vi "read big txt.vi"() -> (2 "selected path":path caption="선택된 경로", 3 "Output":string)   [LabVIEW 2015]
panel:
  out "Output 4":string
  out "Output 3":string
  out "Output 2":string
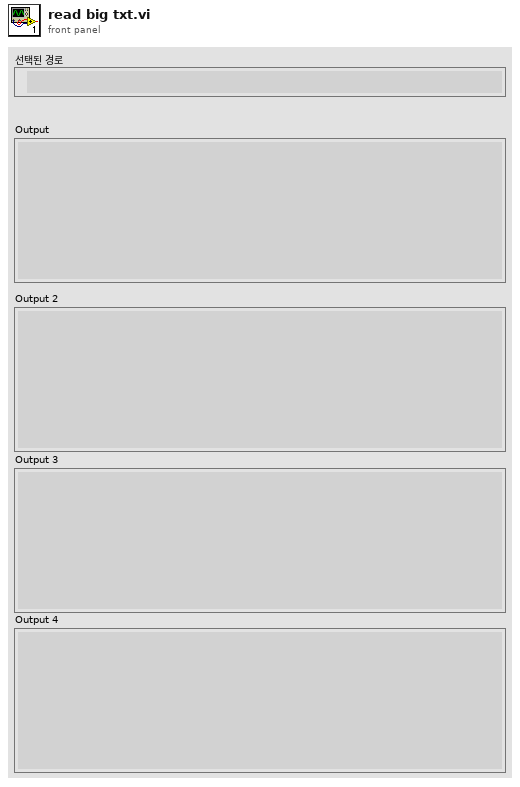
[diagram p1: front panel]
types:
  T1 = enum16{"open", "replace", "create", "open or create", "replace or create", "replace or create with confirmation"}
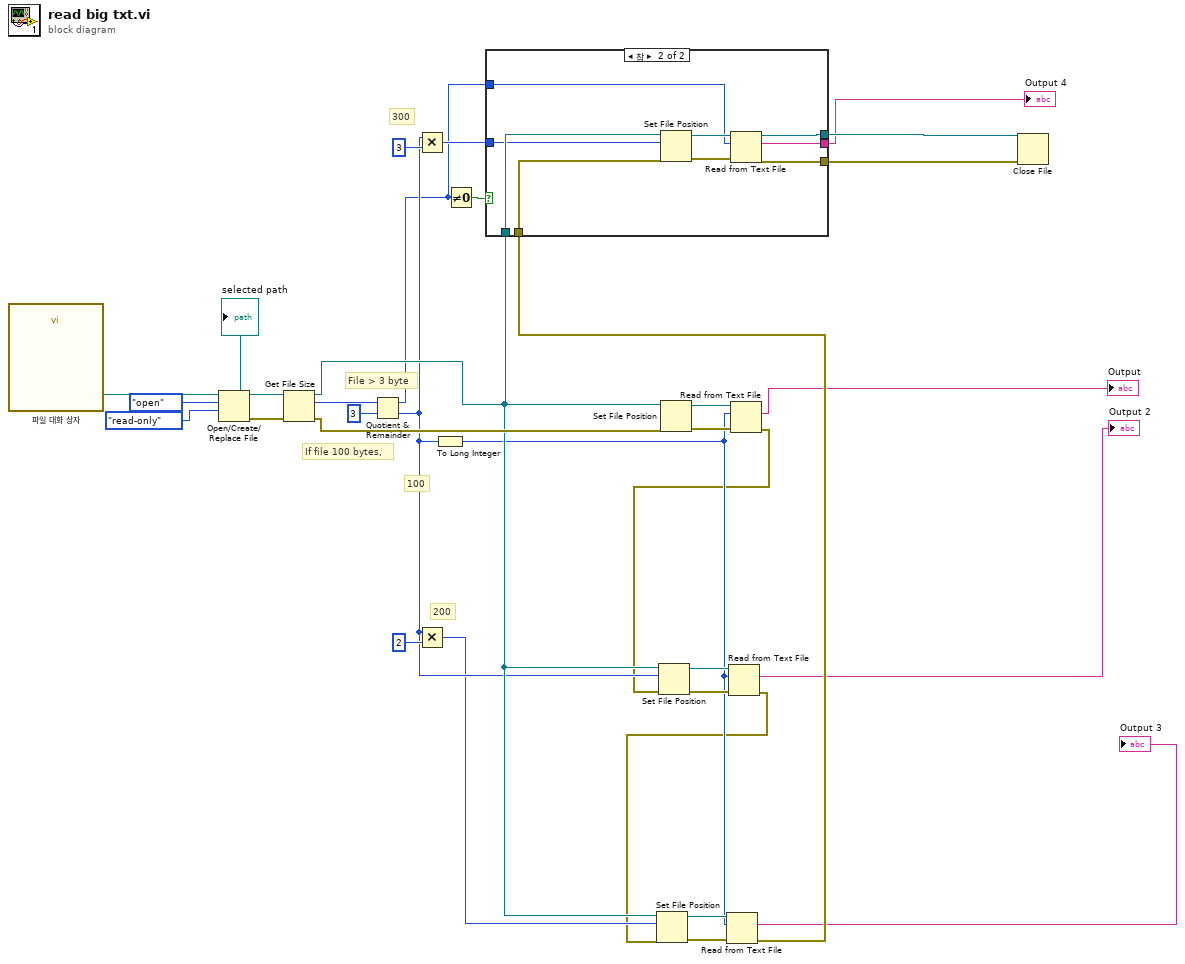
[diagram p0: block diagram]
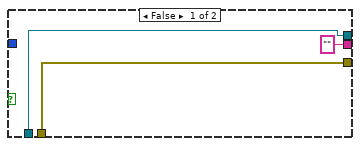
[diagram p2: hidden frame]
diagram:
  # "300"
  # "200"
  # "100"
  # "If file 100 bytes,"
  # "File > 3 byte"
  n1 = call "파일 대화 상자"() -> ("selected path"=w32:path)  [unwired: 12 in, 3 out]
  "selected path" <- w32
  n2 = Open/Create/Replace File(file path (use dialog)=w32, operation (0:open)=T1."open" ("동작(0:open)"), access (0:read/write)=enum16{"read/write", "read-only", "write-only"}."read-only" ("접근(0:읽기/쓰기)")) -> (refnum out=w29:refnum<file>, error out=w28:errorcluster)  [unwired: 3 in, 1 out]
  n3 = Get File Size(file=w29, error in=w28) -> (refnum out=w21:refnum<file>, size (in bytes)=w27:i64, 0:w22:errorcluster)
  n4 = Quotient & Remainder(x=w27, y=i64 3) -> (x-y*floor(x/y)=w10:i64, floor(x/y)=w12:i64)
  n5 = Multiply(x=w12, y=i64 3) -> (x*y=w13:i64)
  n6 = Multiply(x=w12, y=i64 2) -> (x*y=w11:i64)
  n7 = To Long Integer(number=w12) -> (32bit integer=w14:i32)
  n8 = Not Equal To 0?(x=w10) -> (x != 0?=w25:bool)
  n9 = Set File Position(refnum=w21, error in=w22) -> (refnum out=w19:refnum<file>, error out=w20:errorcluster)  [unwired: 2 in]
  n10 = Read from Text File(file (use dialog)=w19, count=w14, error in=w20) -> (text=→"Output":string, error out=w9:errorcluster)  [unwired: 1 in, 2 out]
  n11 = Set File Position(offset (in bytes) (0)=w12, refnum=w21, error in=w9) -> (refnum out=w17:refnum<file>, error out=w18:errorcluster)  [unwired: 1 in]
  n12 = Read from Text File(file (use dialog)=w17, count=w14, error in=w18) -> (text=→"Output 2":string, error out=w8:errorcluster)  [unwired: 1 in, 2 out]
  n13 = Set File Position(offset (in bytes) (0)=w11, refnum=w21, error in=w8) -> (refnum out=w15:refnum<file>, error out=w16:errorcluster)  [unwired: 1 in]
  n14 = Read from Text File(file (use dialog)=w15, count=w14, error in=w16) -> (text=→"Output 3":string, error out=w7:errorcluster)  [unwired: 1 in, 2 out]
  n15 = case shown="참" w25 {
    tunnel: w21 -> [w33 w44]
    tunnel: w7 -> [w34 w43]
    tunnel: w13 -> [_ w40]
    tunnel: w10 -> [_ w39]
    tunnel: ["" w38] -> w1
    tunnel: [w34 w37] -> w6
    tunnel: [w33 w36] -> w5
    frame False {
    }
    frame True {
      n16 = Set File Position(offset (in bytes) (0)=w40, refnum=w44, error in=w43) -> (refnum out=w41:refnum<file>, error out=w42:errorcluster)  [unwired: 1 in]
      n17 = Read from Text File(file (use dialog)=w41, count=w39, error in=w42) -> (refnum out=w36:refnum<file>, text=w38:string, error out=w37:errorcluster)  [unwired: 1 in, 1 out]
    }
  }
  "Output 4" <- w1
  n18 = Close File(refnum=w5, error in=w6) -> ()  [unwired: 2 out]
